vi "Test JSON to Variant (refnum).vi"() -> ()   [LabVIEW 2011]
uses:
  JSON Value/Set from JSON string.vi
  JSON Value/Get as JSON string (pretty).vi
  JSON Value/JSON Value.lvclass
  Variant JSON.lvlib
  Get Polymorphic/JSON GetSet.lvlib
panel:
  out "Equal?":T1
  out "Variant before setting":variant
  out "Variant after setting":variant
  out "JSON String created":string
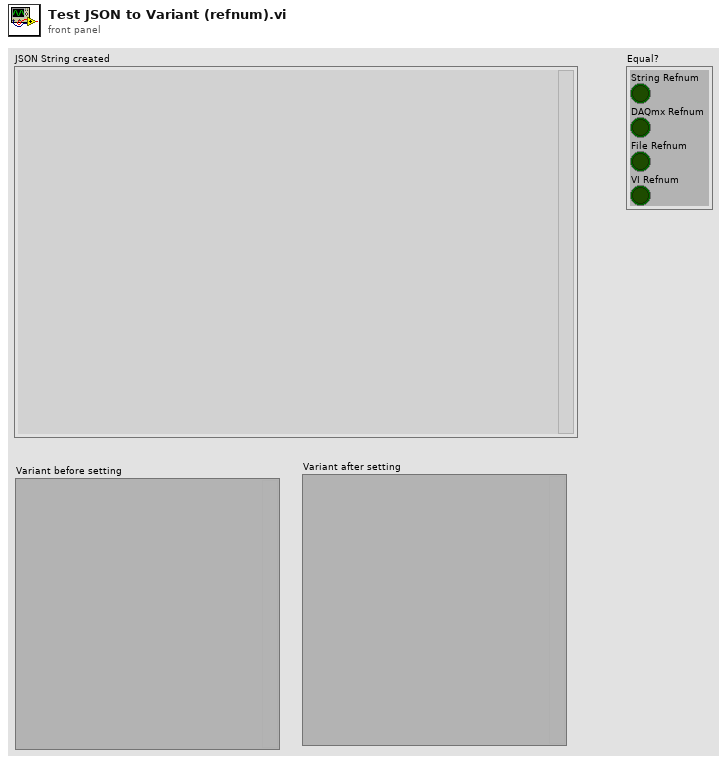
[diagram p1: front panel]
types:
  T1 = cluster{"String Refnum":bool, "DAQmx Refnum":bool, "File Refnum":bool, "VI Refnum":bool}
  T2 = cluster{"String Refnum":refnum<vi>, "DAQmx Refnum":refnum<k21>, "File Refnum":refnum<file>, "VI Refnum":refnum<vi>}
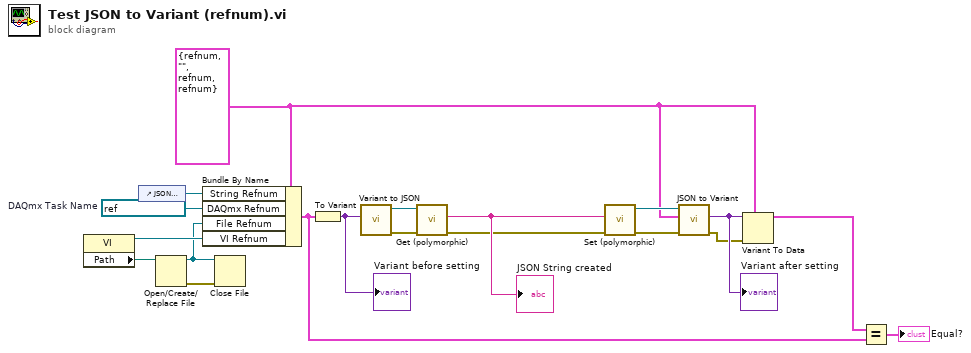
[diagram p0: block diagram]
diagram:
  w4 = T2 {"String Refnum"=refnum, "DAQmx Refnum"="", "File Refnum"=refnum, "VI Refnum"=refnum}
  w10 = refnum<k21> "SampleTask"  # DAQmx Task Name
  n1 = property class="VI"() -> (reference out=w8:refnum<vi>, "Path"=w9:path)  [unwired: 2 in, 1 out]
  n2 = control-ref of="JSON String created"() -> (w11:refnum<vi>)
  n3 = Open/Create/Replace File(file path (use dialog)=w9) -> (refnum out=w2:refnum<file>, error out=w1:errorcluster)  [unwired: 5 in, 1 out]
  n4 = Bundle By Name(cluster=w4, "String Refnum"=w11, "DAQmx Refnum"=w10, "File Refnum"=w2, "VI Refnum"=w8) -> (w5:T2)
  n5 = Close File(refnum=w2, error in=w1) -> ()  [unwired: 2 out]
  n6 = To Variant(anything=w5) -> (Variant=w7:variant)
  "Variant before setting" <- w7
  n7 = call "Variant to JSON.vi"("Variant"=w7) -> ("error out"=w17:errorcluster, "JSON Value out"=w19:refnum<class "JSON Value.lvclass">)  [unwired: 9 in]
  n8 = call-poly "Get (polymorphic).vi"("error in (no error)"=w17, "JSON Value in"=w19) -> ("error out"=w16:errorcluster, "String"=w18:string)  [unwired: 8 in]
  "JSON String created" <- w18
  n9 = call-poly "Set (polymorphic).vi"("error in (no error)"=w16, "JSON stream"=w18) -> ("error out"=w12:errorcluster, "JSON Value out"=w13:refnum<class "JSON Value.lvclass">)  [unwired: 7 in, 1 out]
  n10 = call "JSON to Variant.vi"("error in (no error)"=w12, "Variant (Data Type)"=w4, "JSON Value"=w13) -> ("error out"=w14:errorcluster, "Variant out"=w15:variant)  [unwired: 7 in]
  "Variant after setting" <- w15
  n11 = Variant To Data(error in=w14, type=w4, Variant=w15) -> (data=w6:T2)  [unwired: 1 out]
  n12 = Equal?(x=w6, y=w5) -> (x = y?=→"Equal?":T1)
